vi "HH Scope Control.vi"(6 "Device Outputs in":dbl[](array[numeric]), 8 "error in":errorcluster, 9 "Device Inputs":dbl[](array[numeric]), 10 "DCM Ref":refnum<class "DCM - RT.lvclass">, 11 "HH ADC in":T1={"FIFO Indexes"={"Write"={"Capture Enable"=-1, "Capture Event"=-1, "Capture Length"=-1}, "Read"={"Capture dt [s]"=-1}}, "HH ADC Data"={"Output Array"=[], "New Data"=FALSE}, "Waveform Data"=[], "Waveform Session"=refnum}) -> (0 "error out":errorcluster, 3 "HH ADC out":T1={"FIFO Indexes"={"Write"={"Capture Enable"=-1, "Capture Event"=-1, "Capture Length"=-1}, "Read"={"Capture dt [s]"=-1}}, "HH ADC Data"={"Output Array"=[], "New Data"=FALSE}, "Waveform Data"=[], "Waveform Session"=refnum}, 4 "Device Outputs out":dbl[](array[numeric]))   [LabVIEW 2016, in "DCM Engine.lvlib"]
uses:
  DCM Engine.lvlib
  Shared/Types/HH Scope.ctl
  <vilib>/NI Veristand/Custom Device Waveform API/Multiple Waveforms Write (DBL)/Multiple Waveforms Write (DBL).lvclass
  <vilib>/NI Veristand/Custom Device API/Waveform Data Reference.ctl
  Built/DCM Classes Packed/Pharlap/C/DCM-Classes.lvlibp/DCM/Rev0/RT/DCM - RT.lvclass
  <vilib>/NI Veristand/Custom Device Waveform API/Multiple Waveforms Write (DBL)/NI VeriStand - Close Multiple Waveforms Write Session (DBL).vi
  <vilib>/NI Veristand/Custom Device Waveform API/Multiple Waveforms Write (DBL)/NI VeriStand - Open Multiple Waveforms Write Session (DBL).vi
  Built/DCM Classes Packed/Pharlap/C/DCM-Classes.lvlibp/DCM/HH/RT/DCM - RT - HH.lvlib
  <vilib>/NI Veristand/Custom Device Waveform API/NI_VS Custom Device Waveform API.lvlib
  DCM Shared.lvlib
  <vilib>/NI VeriStand/Custom Device API/Custom Device API.lvlib
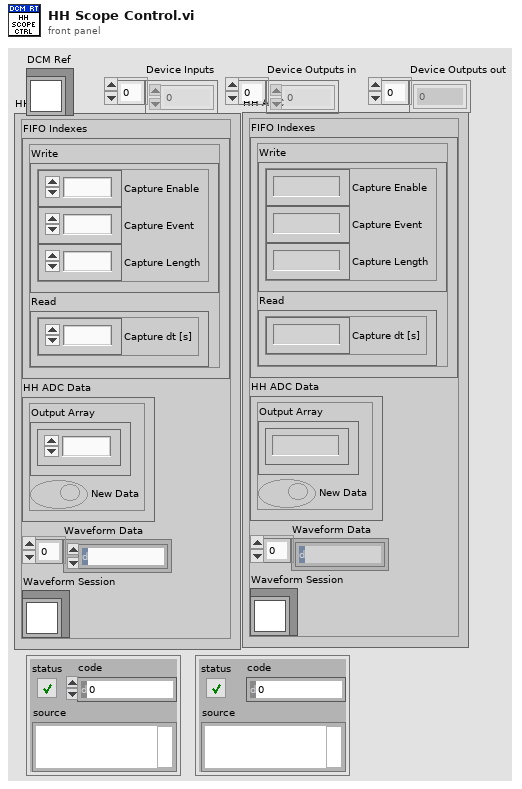
[diagram p1: front panel]
types:
  T1 = typedef "DCM Shared.lvlib/HH Scope.ctl" = cluster{"FIFO Indexes":cluster{"Write":cluster{"Capture Enable":i32, "Capture Event":i32, "Capture Length":i32}, "Read":cluster{"Capture dt [s]":i32}}, "HH ADC Data":cluster{"Output Array":sgl[][], "New Data":bool}, "Waveform Data":T2[], "Waveform Session":refnum<class "Multiple Waveforms Write (DBL).lvclass">}
  T2 = typedef "Custom Device API.lvlib/Waveform Data Reference.ctl" = i32
  T3 = cluster{"Capture Enable":i32, "Capture Event":i32, "Capture Length":i32}
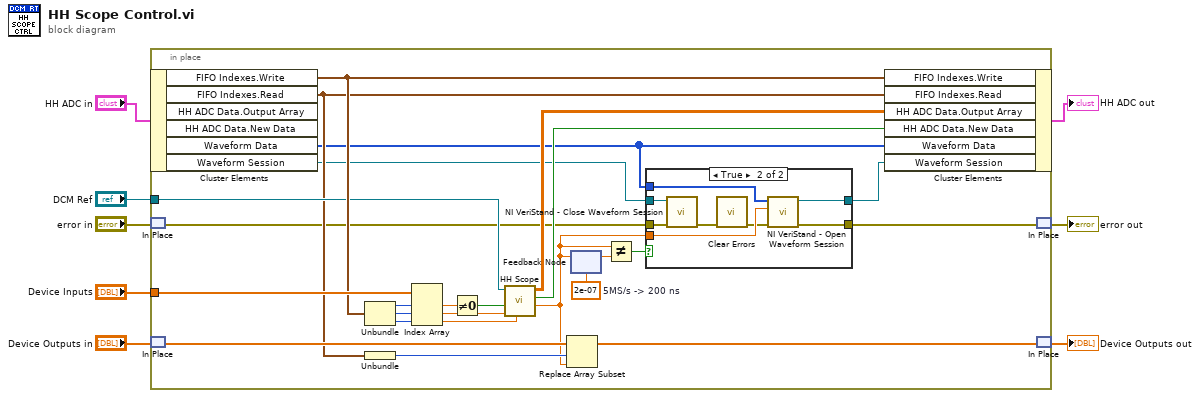
[diagram p0: block diagram]
diagram:
  n1 = in-place {
    in-place-border: "Device Inputs" -> [w33]
    in-place-border: "DCM Ref" -> [w24]
    w9 = 2e-07  # 5MS/s -> 200 ns
    n2 = in-place-cluster #1("HH ADC in") -> ("FIFO Indexes.Write"=w30:T3, "FIFO Indexes.Read"=w21:cluster{"Capture dt [s]":i32}, "Waveform Data"=w10:T2[], "Waveform Session"=w12:refnum<class "Multiple Waveforms Write (DBL).lvclass">)  [unwired: 2 out]
    n3 = in-place-match #2("error in") -> (w15:errorcluster)
    n4 = in-place-match #3("Device Outputs in") -> (w23:dbl[])
    n5 = Unbundle(w30) -> ("Capture Enable"=w32:i32, "Capture Event"=w31:i32, "Capture Length"=w19:i32)
    n6 = Unbundle(w21) -> ("Capture dt [s]"=w20:i32)
    n7 = Index Array(array=w33, index #1=w32, index #2=w31, index #3=w19) -> (element #1=w27:dbl, element #2=w25:dbl, element #3=w18:dbl)
    n8 = Not Equal To 0?(x=w27) -> (x != 0?=w26:bool)
    n9 = call "HH Scope.vi"("HH Scope Length [s]"=w18, "HH Scope Event"=w25, "HH Scope Capture"=w26, "DCM Reference"=w24) -> ("dT [s]"=w11:sgl, "New Data"=w28:bool, "Data"=w29:sgl[][])  [unwired: 4 in, 1 out]
    n10 = Replace Array Subset(array=w23, new element=w11, index=w20) -> (w22:dbl[])
    n11 = feedback #4(w9) -> (w17:dbl)
    n12 = feedback-in #4(w11) -> ()
    n13 = Not Equal?(x=w11, y=w17) -> (x != y?=w16:bool)
    n14 = case shown="True" w16 {
      tunnel: w12 -> [w34 w43]
      tunnel: w15 -> [w35 w42]
      tunnel: [w35 w40] -> w14
      tunnel: [w34 w39] -> w13
      tunnel: w11 -> [_ w38]
      tunnel: w10 -> [_ w37]
      frame False {
      }
      frame True {
        n15 = call-poly <vilib>:"NI VeriStand - Close Waveform Session.vi"("error in (no error)"=w42, "Multiple Waveforms Write Session (DBL)"=w43) -> ("error out"=w41:errorcluster)  [unwired: 9 in]
        n16 = call <vilib>:"Clear Errors.vi"("error in (no error)"=w41) -> ("error out"=w36:errorcluster)  [unwired: 5 in, 1 out]
        n17 = call-poly <vilib>:"NI VeriStand - Open Waveform Session.vi"("error in (no error)"=w36, "dt"=w38, "DBL Waveform Data References"=w37) -> ("error out"=w40:errorcluster, "Multiple Waveforms Write Session (DBL)"=w39:refnum<class "Multiple Waveforms Write (DBL).lvclass">)  [unwired: 7 in]
      }
    }
    n18 = in-place-cluster #1("FIFO Indexes.Write"=w30, "FIFO Indexes.Read"=w21, "HH ADC Data.Output Array"=w29, "HH ADC Data.New Data"=w28, "Waveform Data"=w10, "Waveform Session"=w13) -> (→"HH ADC out":T1)
    n19 = in-place-match #2(w14) -> (→"error out":errorcluster)
    n20 = in-place-match #3(w22) -> (→"Device Outputs out":dbl[])
  }
